vi "Unflatten Weather Report.vi"(10 "String":string="{\"Headline\":{\"EffectiveDate\":\"2017-10-13T07:00:00+05:30\",\"EffectiveEpochDate\":1507858200,\"Severity\":7,\"Text\":\"Very warm Friday\",\"Category\":\"heat\",\"EndDate\":\"2017-10-13T19:00:00+05:30\",\"EndEpochDate\":1507901400,\"MobileLink\":\"http://m.accuweather.com/en/in/ghaziabad/206683/extended-weather-forecast/206683?lang=en-us\",\"Link\":\"http://www.accuweather.com/en/in/ghaziabad/206683/daily-weather-forecast/206683?lang=en-us\"},\"DailyForecasts\":[{\"Date\":\"2017-10-12T07:00:00+05:30\",\"EpochDate\":1507771800,\"Temperature\":{\"Minimum\":{\"Value\":72.0,\"Unit\":\"F\",\"UnitType\":18},\"Maximum\":{\"Value\":95.0,\"Unit\":\"F\",\"UnitType\":18}},\"Day\":{\"Icon\":1,\"IconPhrase\":\"Sunny\"},\"Night\":{\"Icon\":33,\"IconPhrase\":\"Clear\"},\"Sources\":[\"AccuWeather\"],\"MobileLink\":\"http://m.accuweather.com/en/in/ghaziabad/206683/daily-weather-forecast/206683?day=1&lang=en-us\",\"Link\":\"http://www.accuweather.com/en/in/ghaziabad/206683/daily-weather-forecast/206683?day=1&lang=en-us\"},{\"Date\":\"2017-10-13T07:00:00+05:30\",\"EpochDate\":1507858200,\"Temperature\":{\"Minimum\":{\"Value\":70.0,\"Unit\":\"F\",\"UnitType\":18},\"Maximum\":{\"Value\":96.0,\"Unit\":\"F\",\"UnitType\":18}},\"Day\":{\"Icon\":1,\"IconPhrase\":\"Sunny\"},\"Night\":{\"Icon\":33,\"IconPhrase\":\"Clear\"},\"Sources\":[\"AccuWeather\"],\"MobileLink\":\"http://m.accuweather.com/en/in/ghaziabad/206683/daily-weather-forecast/206683?day=2&lang=en-us\",\"Link\":\"http://www.accuweather.com/en/in/ghaziabad/206683/daily-weather-forecast/206683?day=2&lang=en-us\"},{\"Date\":\"2017-10-14T07:00:00+05:30\",\"EpochDate\":1507944600,\"Temperature\":{\"Minimum\":{\"Value\":69.0,\"Unit\":\"F\",\"UnitType\":18},\"Maximum\":{\"Value\":97.0,\"Unit\":\"F\",\"UnitType\":18}},\"Day\":{\"Icon\":1,\"IconPhrase\":\"Sunny\"},\"Night\":{\"Icon\":33,\"IconPhrase\":\"Clear\"},\"Sources\":[\"AccuWeather\"],\"MobileLink\":\"http://m.accuweather.com/en/in/ghaziabad/206683/daily-weather-forecast/206683?day=3&lang=en-us\",\"Link\":\"http://www.accuweather.com/en/in/ghaziabad/206683/daily-weather-forecast/206683?day=3&lang=en-us\"},{\"Date\":\"2017-10-15T07:00:00+05:30\",\"EpochDate\":1508031000,\"Temperature\":{\"Minimum\":{\"Value\":69.0,\"Unit\":\"F\",\"UnitType\":18},\"Maximum\":{\"Value\":97.0,\"Unit\":\"F\",\"UnitType\":18}},\"Day\":{\"Icon\":1,\"IconPhrase\":\"Sunny\"},\"Night\":{\"Icon\":33,\"IconPhrase\":\"Clear\"},\"Sources\":[\"AccuWeather\"],\"MobileLink\":\"http://m.accuweather.com/en/in/ghaziabad/206683/daily-weather-forecast/206683?day=4&lang=en-us\",\"Link\":\"http://www.accuweather.com/en/in/ghaziabad/206683/daily-weather-forecast/206683?day=4&lang=en-us\"},{\"Date\":\"2017-10-16T07:00:00+05:30\",\"EpochDate\":1508117400,\"Temperature\":{\"Minimum\":{\"Value\":68.0,\"Unit\":\"F\",\"UnitType\":18},\"Maximum\":{\"Value\":97.0,\"Unit\":\"F\",\"UnitType\":18}},\"Day\":{\"Icon\":1,\"IconPhrase\":\"Sunny\"},\"Night\":{\"Icon\":33,\"IconPhrase\":\"Clear\"},\"Sources\":[\"AccuWeather\"],\"MobileLink\":\"http://m.accuweather.com/en/in/ghaziabad/206683/daily-weather-forecast/206683?day=5&lang=en-us\",\"Link\":\"http://www.accuweather.com/en/in/ghaziabad/206683/daily-weather-forecast/206683?day=5&lang=en-us\"}]}") -> (2 "Array":T1(array[cluster]))   [LabVIEW 2013]
uses:
  <vilib>/Utility/file.llb/Write To Spreadsheet File (string).vi
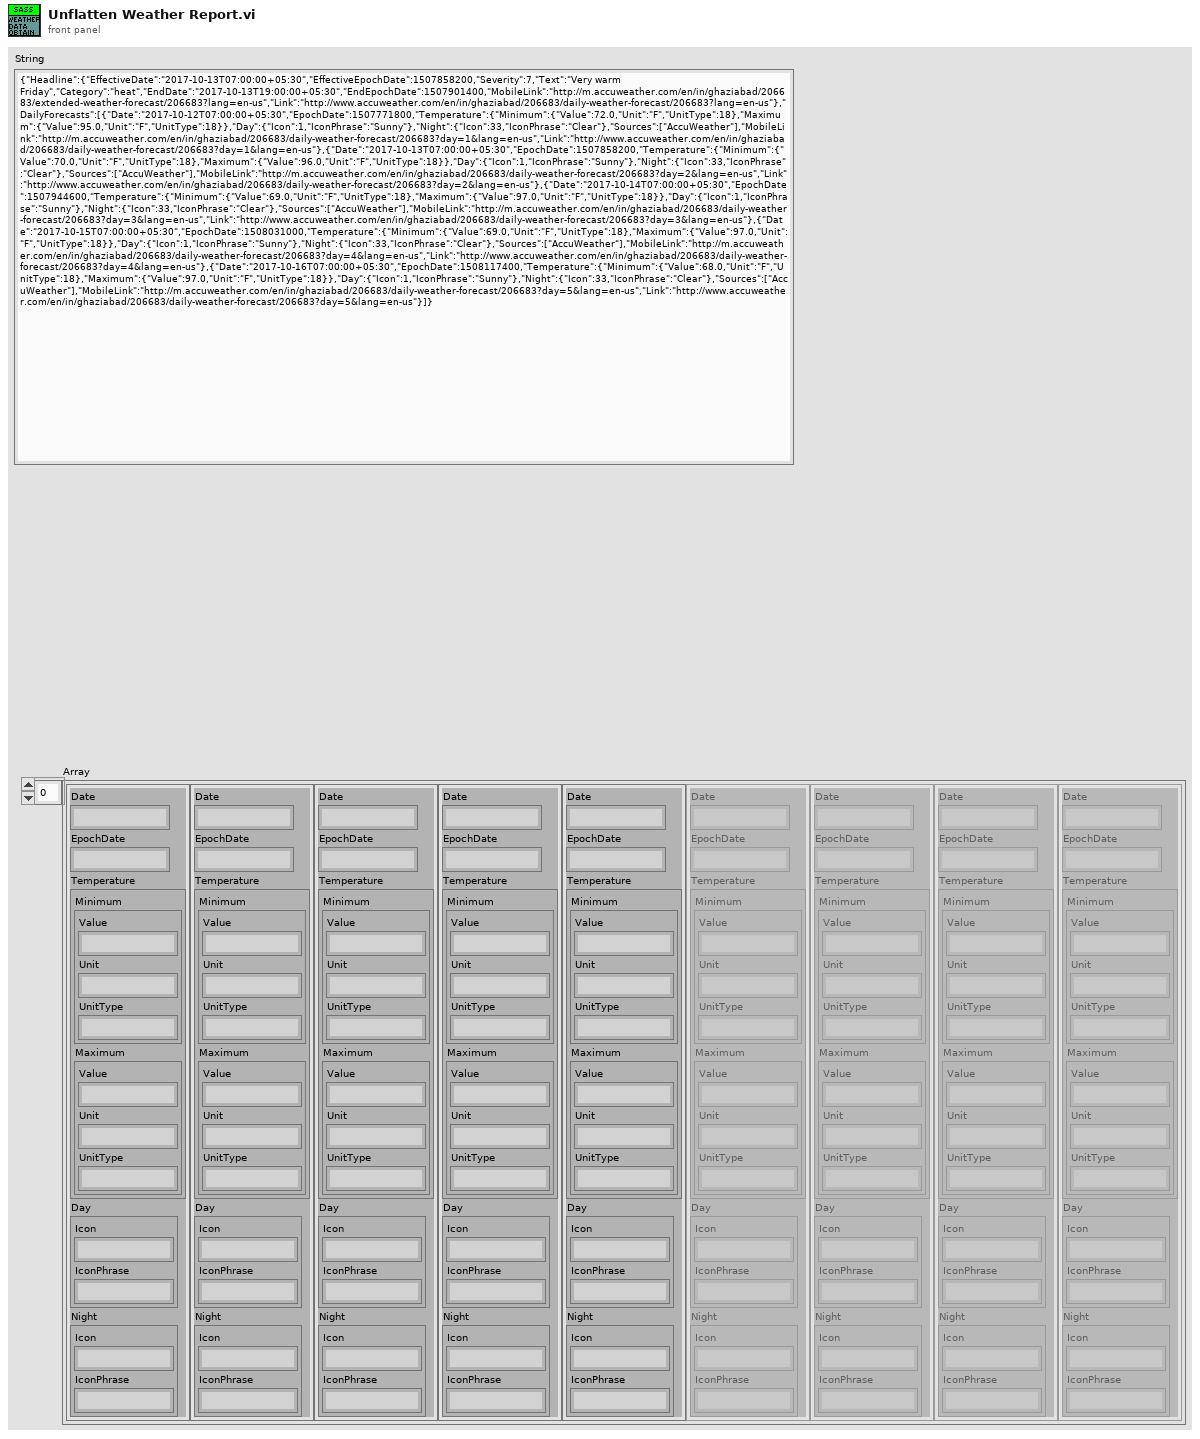
[diagram p1: front panel]
types:
  T1 = cluster{"Date":string, "EpochDate":string, "Temperature":cluster{"Minimum":cluster{"Value":string, "Unit":string, "UnitType":string}, "Maximum":cluster{"Value":string, "Unit":string, "UnitType":string}}, "Day":cluster{"Icon":string, "IconPhrase":string}, "Night":cluster{"Icon":string, "IconPhrase":string}}[]
  T2 = cluster{"Date":string, "EpochDate":string, "Temperature":cluster{"Minimum":cluster{"Value":string, "Unit":string, "UnitType":string}, "Maximum":cluster{"Value":string, "Unit":string, "UnitType":string}}, "Day":cluster{"Icon":string, "IconPhrase":string}, "Night":cluster{"Icon":string, "IconPhrase":string}}
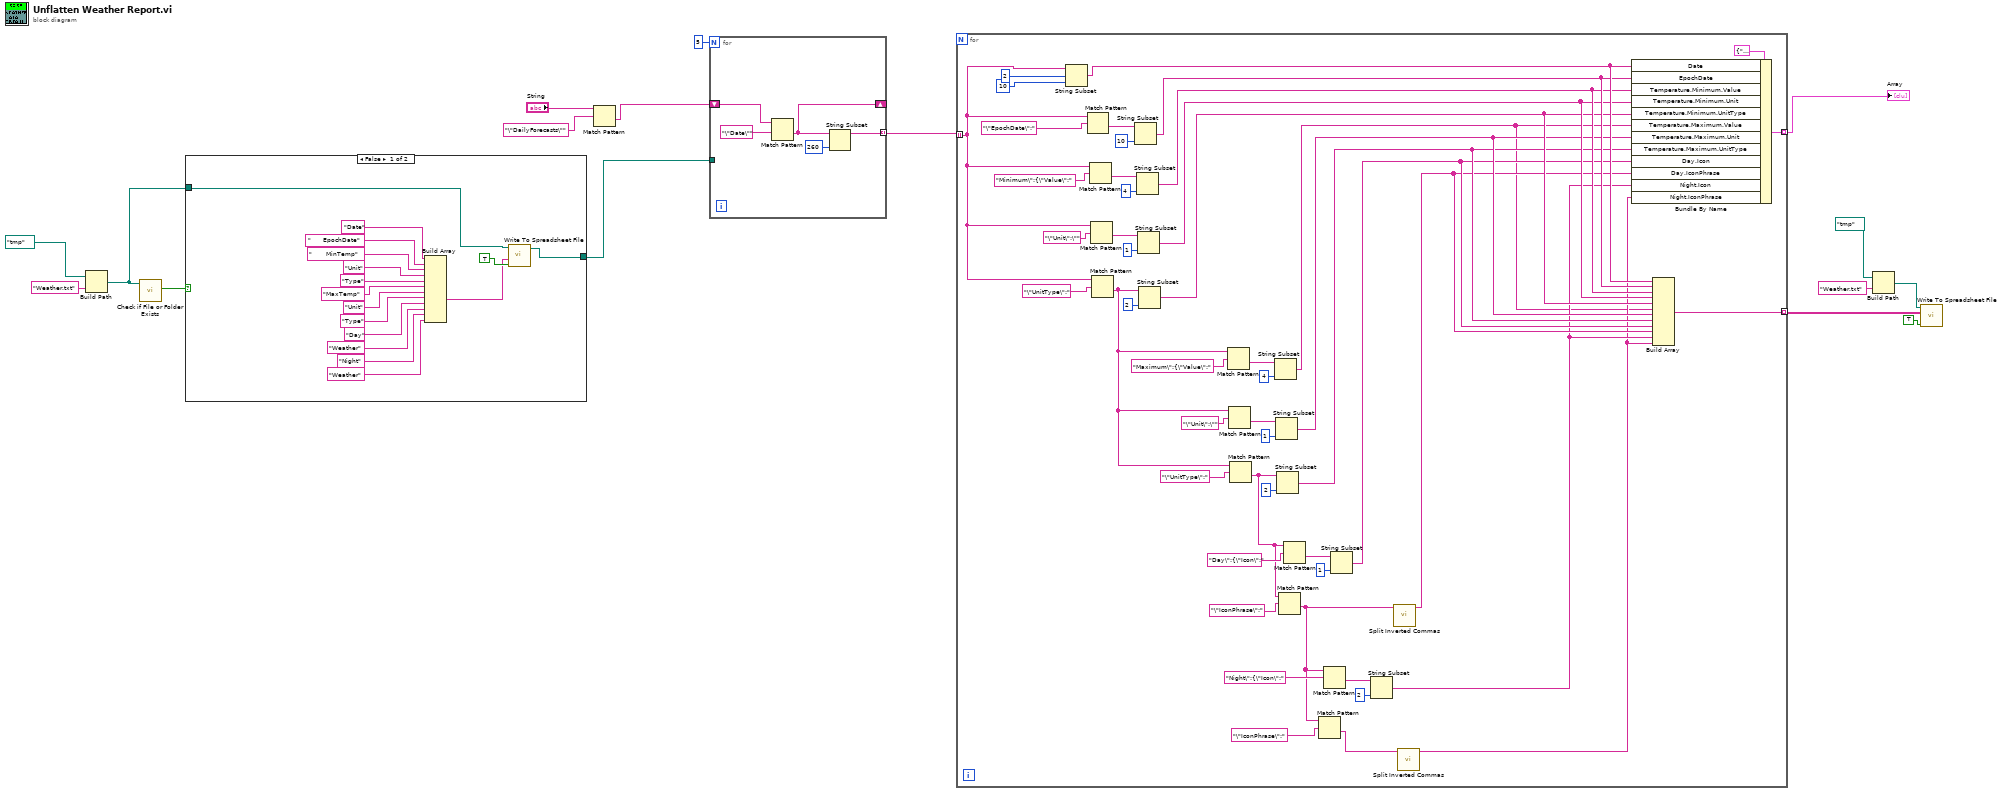
[diagram p0: block diagram]
diagram:
  n1 = Build Path(base path=path "/tmp", name or relative path="Weather.txt") -> (appended path=w7:path)
  n2 = call <vilib>:"Check if File or Folder Exists.vi"("path"=w7) -> ("file or folder exists?"=w3:bool)  [unwired: 8 in, 2 out]
  n3 = case shown="False" w3 {
    tunnel: w7 -> [w19 _]
    tunnel: [w17 _] -> w5
    frame False {
      n4 = Build Array("Date" ("regular expression"), "      EpochDate" ("regular expression"), "       MinTemp" ("regular expression"), "Unit" ("regular expression"), "Type" ("regular expression"), "MaxTemp" ("regular expression"), "Unit" ("regular expression"), "Type" ("regular expression"), "Day" ("regular expression"), "Weather" ("regular expression"), "Night" ("regular expression"), "Weather" ("regular expression")) -> (w18:string[])
      n5 = call-poly <vilib>:"Write To Spreadsheet File.vi"("append to file? (new file:F)"=TRUE ("append to file? (F)"), "1D data"=w18, "file path (dialog if empty)"=w19) -> ("new file path (Not A Path if cancelled)"=w17:path)  [unwired: 5 in]
    }
    frame True {
    }
  }
  n6 = Match Pattern(string="String", regular expression="\"DailyForecasts\"") -> (after substring=w14:string)  [unwired: 1 in, 3 out]
  n7 = for {
    N: 5 -> [_]
    tunnel: [w34] -> w12 mode=indexing
    shift-right: [w35] -> _
    shift-left: w14 -> [w37]
    tunnel: w5 -> [_]
    n8 = Match Pattern(string=w37, regular expression="\"Date\"") -> (after substring=w35:string)  [unwired: 1 in, 3 out]
    n9 = String Subset(string=w35, length (rest)=260 ("length (rest)")) -> (substring=w34:string)  [unwired: 1 in]
  }
  n10 = for {
    tunnel: w12 -> [w72] mode=indexing
    tunnel: [w62] -> w11 mode=indexing
    tunnel: [w39] -> w4 mode=indexing
    n11 = String Subset(string=w72, offset (0)=2, length (rest)=10 ("length (rest)")) -> (substring=w50:string)
    n12 = Match Pattern(string=w72, regular expression="\"EpochDate\":") -> (after substring=w82:string)  [unwired: 1 in, 3 out]
    n13 = Match Pattern(string=w72, regular expression="Minimum\":{\"Value\":") -> (after substring=w79:string)  [unwired: 1 in, 3 out]
    n14 = Match Pattern(string=w72, regular expression="\"Unit\":\"") -> (after substring=w76:string)  [unwired: 1 in, 3 out]
    n15 = Match Pattern(string=w72, regular expression="\"UnitType\":") -> (after substring=w64:string)  [unwired: 1 in, 3 out]
    n16 = String Subset(string=w82, length (rest)=10 ("length (rest)")) -> (substring=w49:string)  [unwired: 1 in]
    n17 = String Subset(string=w79, length (rest)=4 ("length (rest)")) -> (substring=w48:string)  [unwired: 1 in]
    n18 = String Subset(string=w76, length (rest)=1 ("length (rest)")) -> (substring=w47:string)  [unwired: 1 in]
    n19 = String Subset(string=w64, length (rest)=2 ("length (rest)")) -> (substring=w46:string)  [unwired: 1 in]
    n20 = Match Pattern(string=w64, regular expression="Maximum\":{\"Value\":") -> (after substring=w63:string)  [unwired: 1 in, 3 out]
    n21 = Match Pattern(string=w64, regular expression="\"Unit\":\"") -> (after substring=w68:string)  [unwired: 1 in, 3 out]
    n22 = Match Pattern(string=w64, regular expression="\"UnitType\":") -> (after substring=w57:string)  [unwired: 1 in, 3 out]
    n23 = String Subset(string=w63, length (rest)=4 ("length (rest)")) -> (substring=w38:string)  [unwired: 1 in]
    n24 = String Subset(string=w68, length (rest)=1 ("length (rest)")) -> (substring=w45:string)  [unwired: 1 in]
    n25 = String Subset(string=w57, length (rest)=2 ("length (rest)")) -> (substring=w44:string)  [unwired: 1 in]
    n26 = Match Pattern(string=w57, regular expression="\"IconPhrase\":") -> (after substring=w51:string)  [unwired: 1 in, 3 out]
    n27 = Match Pattern(string=w57, regular expression="Day\":{\"Icon\":") -> (after substring=w61:string)  [unwired: 1 in, 3 out]
    n28 = Match Pattern(string=w51, regular expression="\"IconPhrase\":") -> (after substring=w56:string)  [unwired: 1 in, 3 out]
    n29 = Match Pattern(string=w51, regular expression="Night\":{\"Icon\":") -> (after substring=w52:string)  [unwired: 1 in, 3 out]
    n30 = String Subset(string=w61, length (rest)=1 ("length (rest)")) -> (substring=w43:string)  [unwired: 1 in]
    n31 = String Subset(string=w52, length (rest)=2 ("length (rest)")) -> (substring=w41:string)  [unwired: 1 in]
    n32 = call "Split Inverted Commas.vi"("String in"=w51) -> ("String out"=w42:string)  [unwired: 10 in]
    n33 = call "Split Inverted Commas.vi"("String in"=w56) -> ("String out"=w40:string)  [unwired: 10 in]
    n34 = Bundle By Name(cluster=T2 {"Date"="", "EpochDate"="", "Temperature"={"Minimum"={"Value"="", "Unit"="", "UnitType"=""}, "Maximum"={"Value"="", "Unit"="", "UnitType"=""}}, "Day"={"Icon"="", "IconPhrase"=""}, "Night"={"Icon"="", "IconPhrase"=""}}, "Date"=w50, "EpochDate"=w49, "Temperature.Minimum.Value"=w48, "Temperature.Minimum.Unit"=w47, "Temperature.Minimum.UnitType"=w46, "Temperature.Maximum.Value"=w38, "Temperature.Maximum.Unit"=w45, "Temperature.Maximum.UnitType"=w44, "Day.Icon"=w43, "Day.IconPhrase"=w42, "Night.Icon"=w41, "Night.IconPhrase"=w40) -> (w62:T2)
    n35 = Build Array(w50, w49, w48, w47, w46, w38, w45, w44, w43, w42, w41, w40) -> (w39:string[])
  }
  "Array" <- w11
  n36 = Build Path(base path=path "/tmp", name or relative path="Weather.txt") -> (appended path=w9:path)
  n37 = call-poly <vilib>:"Write To Spreadsheet File.vi"("append to file? (new file:F)"=TRUE ("append to file? (F)"), "2D data"=w4, "file path (dialog if empty)"=w9) -> ()  [unwired: 5 in, 1 out]
